vi "Example Configuration.vi"() -> ()   [LabVIEW 2013]
uses:
  C:/tf/play/labview/Tinkerforge.dll
  Tinkerforge.dll
panel:
  in  "uid":string="63oL6P"
  in  "port":i32=4223
  in  "host":string="localhost"
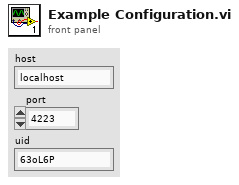
[diagram p1: front panel]
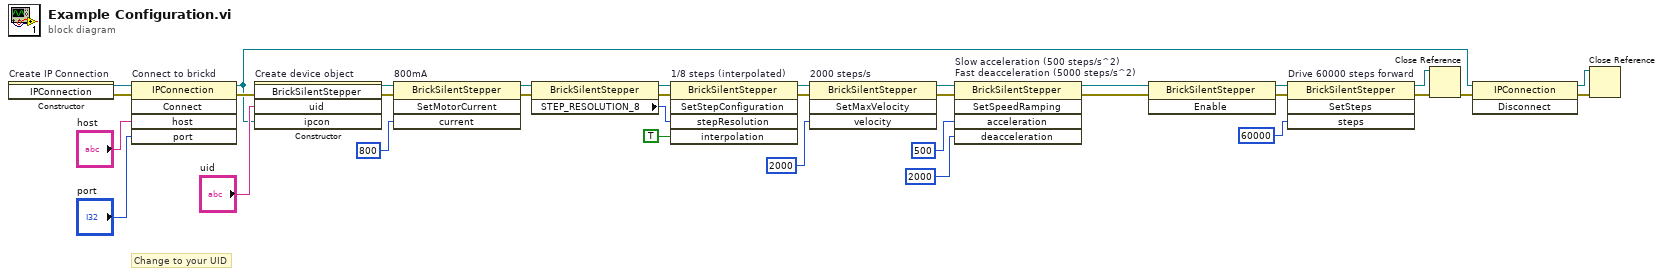
[diagram p0: block diagram]
diagram:
  # "Change to your UID"
  n1 = constructor on="Create IP Connection" class="IPConnection"() -> (reference out=w33:refnum<k24>, error out=w7:errorcluster)  [unwired: 3 in, 1 out]
  n2 = invoke on="Connect to brickd" class="IPConnection" method="Connect"(reference=w33, error in=w7, "host"="host", "port"="port") -> (reference out=w24:refnum<k24>, error out=w29:errorcluster)  [unwired: 1 in, 3 out]
  n3 = constructor on="Create device object" class="BrickSilentStepper"(error in=w29, "uid"="uid", "ipcon"=w24) -> (reference out=w27:refnum<k24>, error out=w28:errorcluster)  [unwired: 2 in, 3 out]
  n4 = invoke on="800mA" class="BrickSilentStepper" method="SetMotorCurrent"(reference=w27, error in=w28, "current"=800) -> (reference out=w5:refnum<k24>, error out=w4:errorcluster)  [unwired: 1 in, 2 out]
  n5 = property class="BrickSilentStepper"(reference=w5, error in=w4) -> (reference out=w6:refnum<k24>, error out=w3:errorcluster, "STEP_RESOLUTION_8"=w2:u8)
  n6 = invoke on="1/8 steps (interpolated)" class="BrickSilentStepper" method="SetStepConfiguration"(reference=w6, error in=w3, "stepResolution"=w2, "interpolation"=TRUE) -> (reference out=w20:refnum<k24>, error out=w21:errorcluster)  [unwired: 1 in, 3 out]
  n7 = invoke on="2000 steps/s" class="BrickSilentStepper" method="SetMaxVelocity"(reference=w20, error in=w21, "velocity"=2000) -> (reference out=w17:refnum<k24>, error out=w18:errorcluster)  [unwired: 1 in, 2 out]
  n8 = invoke on="Slow acceleration (500 steps/s^2)\nFast deacceleration (5000 steps/s^2)" class="BrickSilentStepper" method="SetSpeedRamping"(reference=w17, error in=w18, "acceleration"=500, "deacceleration"=2000) -> (reference out=w13:refnum<k24>, error out=w14:errorcluster)  [unwired: 1 in, 3 out]
  n9 = invoke class="BrickSilentStepper" method="Enable"(reference=w13, error in=w14) -> (reference out=w11:refnum<k24>, error out=w12:errorcluster)  [unwired: 1 in, 1 out]
  n10 = invoke on="Drive 60000 steps forward" class="BrickSilentStepper" method="SetSteps"(reference=w11, error in=w12, "steps"=60000) -> (reference out=w8:refnum<k24>, error out=w9:errorcluster)  [unwired: 1 in, 2 out]
  n11 = Close Reference(reference=w8, error in (no error)=w9) -> (error out=w26:errorcluster)
  n12 = invoke class="IPConnection" method="Disconnect"(reference=w24, error in=w26) -> (reference out=w23:refnum<k24>, error out=w25:errorcluster)  [unwired: 1 in, 1 out]
  n13 = Close Reference(reference=w23, error in (no error)=w25) -> ()  [unwired: 1 out]
